vi "pco.camera_Live_ConvertSettings_Example_IMAQ.vi"() -> ()   [LabVIEW 2020]
doc: "A short program to demonstrate the fundamentals of control and image acquision with the pco.camera series. The program records a sequence of images, with \"live\" updating, until the \"StopRecording\" button is pressed. Use ctrl-H for more help on the individual controls and indicators.\n\nCopyright 2004, 2010 The Cooke Corporation."
uses:
  Camera.lvclass
  TimingControl.lvlib
panel:
  in  "settingsChanged":bool
  in  "Trigger":bool
  in  "LUT File":path
  in  "data_format":T1(ring)=enum."RGBA8"
  out "Image":T2(plugin-control)
  in  "Auto Range":bool
  out "rawImage":u16[][](array[numeric])
  in  "iContrast [%]":i32 min=-100 max=99 step=1
  in  "Gamma":dbl=1.0 min=0.01 max=10.0 step=0.01 format="%.2f"
  in  "whiteBalance":bool
  in  "iScale_max":u16=60000 step=1
  in  "iScale_min":u16=200 step=1
  in  "Image Index":u32 max=9
  out "Recorded Images":u32
  in  "TriggerMode":T3(ring)
  in  "Quit":bool
  out "Error":errorcluster {"code" format="%x"}
  in  "Stop Record":bool
  out "Recording On":bool
  in  "roiY1":u64=2 min=1 max=2160 step=1
  in  "roiX1":u64=2 min=1 max=2560 step=1
  in  "roiY0":u64=1 min=1 max=2159 step=1
  in  "roiX0":u64=1 min=1 max=2559 step=1
  out "Image Height":u64
  out "Image Width":u64
  in  "dwImgCount":u32=10 caption="Required Number of Images" max=2397
  in  "Exposure Time [s]":dbl=0.010000000000000002 min=0.0005 max=2.0 step=0.001
  # "This example demonstrates the image acquisition with one camera in ring buffer mode together with a live display of the latest images during record. After record is stopped, the images can be addressed by index.\nAdditionally the image convert settings can be adjusted at any time\nNote that this example will not be fail save, i.e. doesnt react on errors, just handles them forward to the end\n\nUsage:\nSelect your required image count and the camera setup before you start the program.\nOnce started, the camera class will be initialized and images will be recorded and displayed automatically\nYou can stop the images by pressing stop record.\nAfter stopped, the image at the selected index will be read out\nTo finish the program click on quit application, this will force an exit of the camera class\nYou can change your required ROI after and also during the record."
  # "pco.labview"
  # "Camera Setup"
  # "Recording Control"
  # "Parameters for image readout"
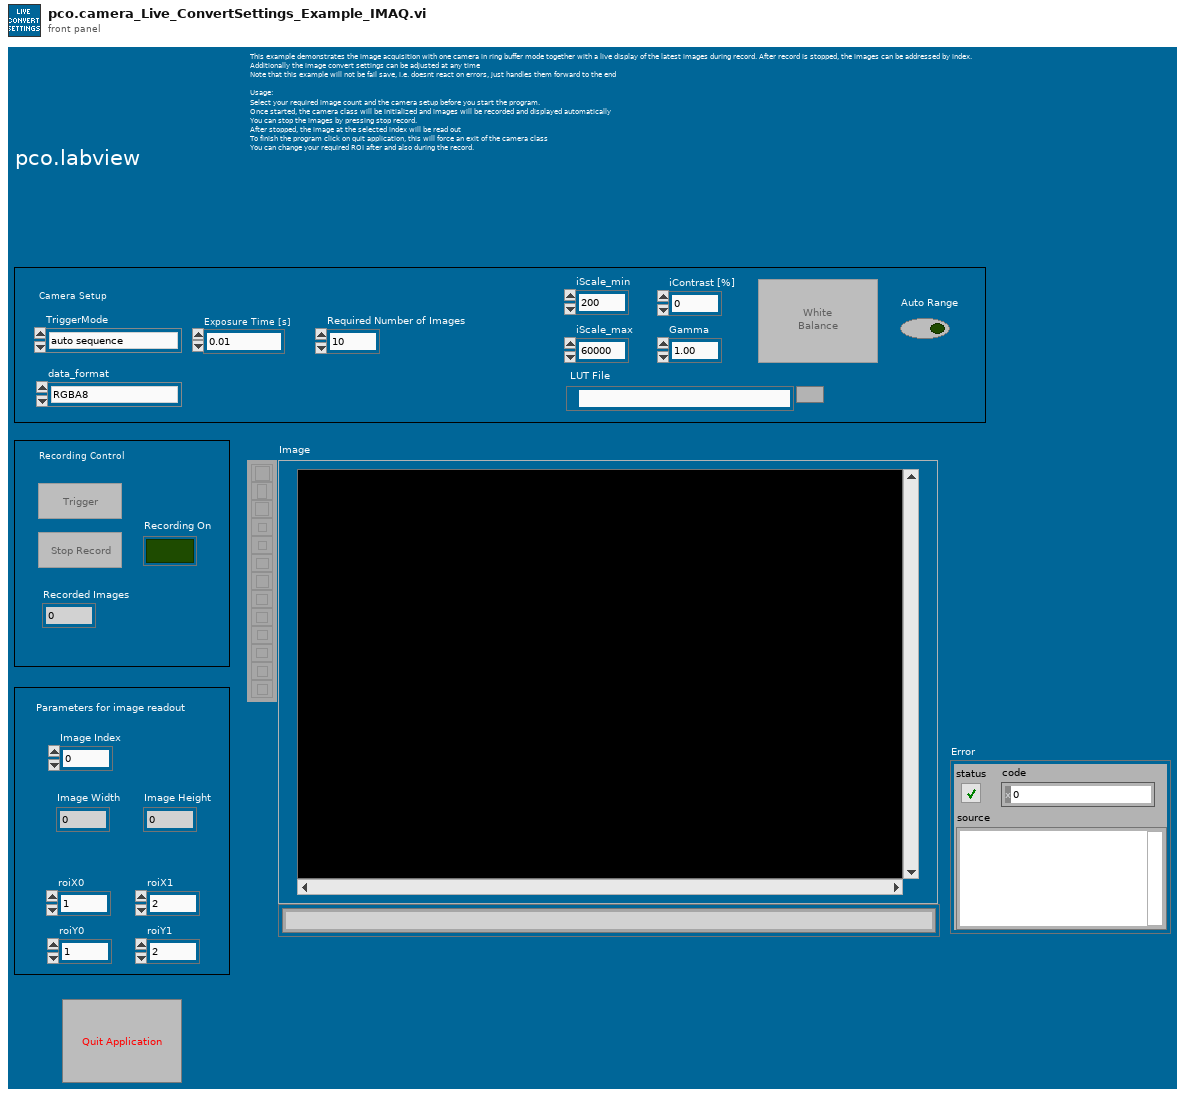
[diagram p1: front panel]
types:
  T1 = enum16{"Undefined", "Mono8", "Mono16", "BGRA8", "RGBA8", "BGRA16", "RGBA16", "CompressedMono8"}
  T2 = typedef "IMAQ Image.ctl" = refnum<image>
  T3 = enum16{"auto sequence", "software trigger", "external exposure start", "external exposure control"}
  T4 = enum16{"sequence", "sequence non blocking", "ring buffer", "fifo", "sequence_dpcore", "sequence_non_blocking_dpcore", "ring_buffer_dpcore", "fifo_dpcore", "tif", "multitif", "pcoraw", "b16", "dicom", "multidicom"}
  T5 = enum8{"Enabled", "Disabled", "Disabled and Grayed Out"}
  T6 = cluster{"serial":u32, "type":u16, "sub_type":u16, "interface_type":u16, "bit_resolution":u16, "min_exposure_time_s":dbl, "max_exposure_time_s":dbl, "min_exposure_step_s":dbl, "min_delay_time_s":dbl, "max_delay_time_s":dbl, "min_delay_step_s":dbl, "min_width":u64, "min_height":u64, "max_width":u64, "max_height":u64, "roi_step_horz":u64, "roi_step_vert":u64, "roi_symmetric_horz":bool, "roi_symmetric_vert":bool, "has_timestamp_mode":bool, "has_timestamp_mode_ascii_only":bool, "pixelrate_vec":u32[], "has_acquire_mode":bool, "has_ext_acquire_mode":bool, "has_metadata_mode":bool, "has_ram":bool, "binning_horz_vec":u16[], "binning_vert_vec":u16[]}
  T7 = typedef "Image Type" = u32
  T8 = typedef "Camera.lvclass/binning.ctl" = cluster{"vert":u16, "horz":u16}
  T9 = cluster{"exposure_time_s":dbl, "delay_time_s":dbl, "roi":cluster{"x0":u64, "y0":u64, "x1":u64, "y1":u64}, "timestamp_mode":u16, "pixelrate":u32, "trigger_mode":u16, "acquire_mode":u16, "metadata_mode":u16, "noisefilter_mode":u16, "binning":T8}
  T10 = cluster{"sharpen":bool, "adaptive_sharpen":bool, "flip_vertical":bool, "auto_minmax":bool, "min_limit":u16, "max_limit":u16, "gamma":dbl, "contrast":i32, "pco_debayer_algorithm":bool, "color_temperature":i32, "color_saturation":i32, "color_vibrance":i32, "color_tint":i32, "lut_file":path}
  T11 = cluster{"Plane 4 (alpha)":u16, "Plane 1 (Red)":u16, "Plane 2 (Green)":u16, "Plane 3 (Blue)":u16}[][]
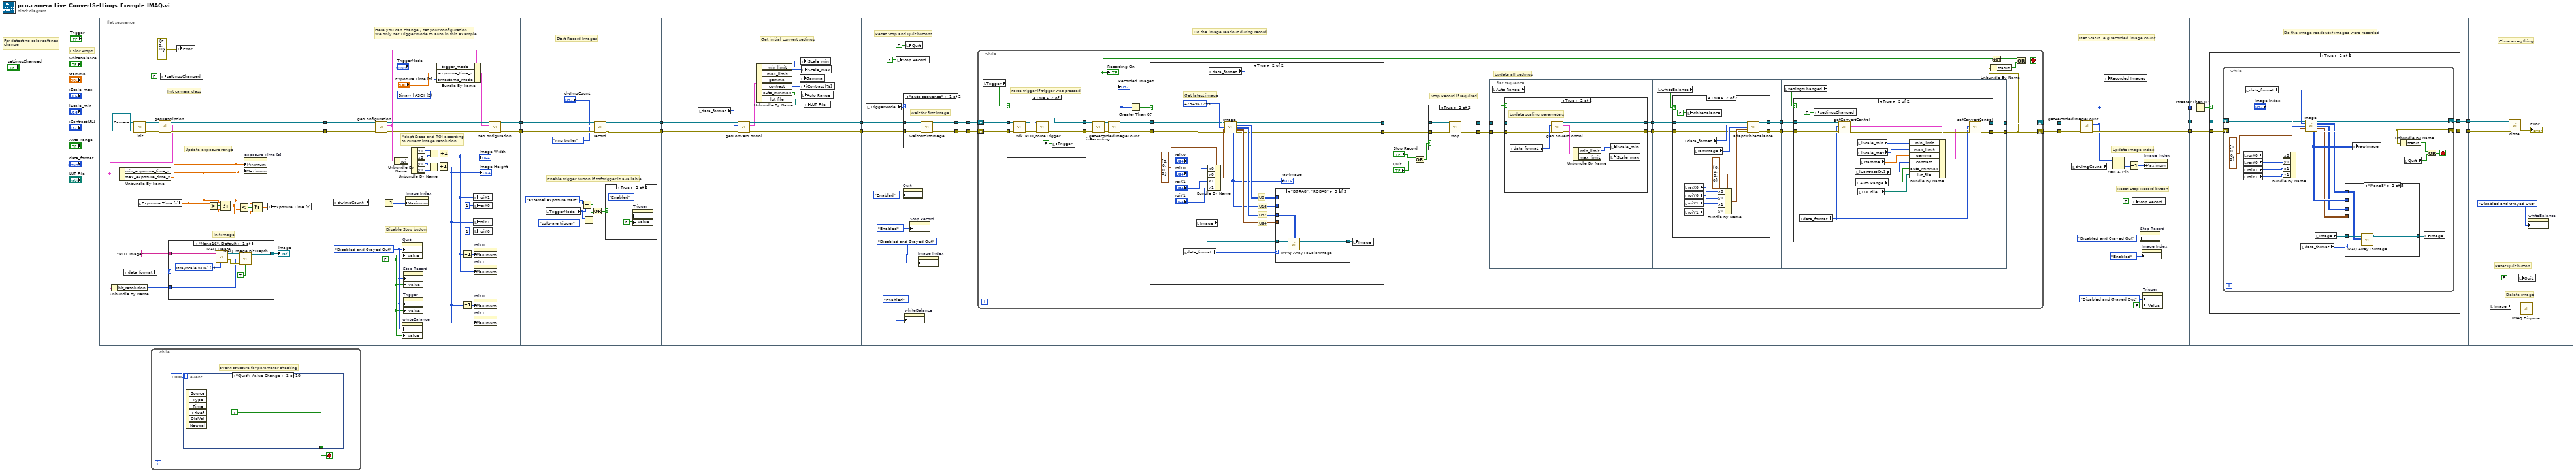
[diagram p0: block diagram]
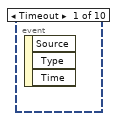
[diagram p2: hidden frame]
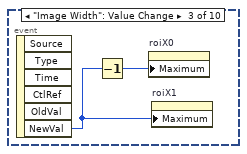
[diagram p3: hidden frame]
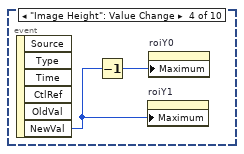
[diagram p4: hidden frame]
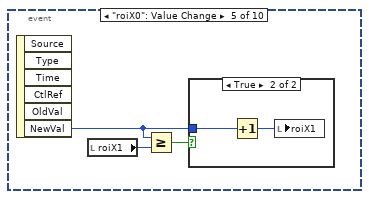
[diagram p5: hidden frame]
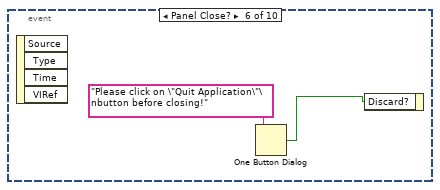
[diagram p7: hidden frame]
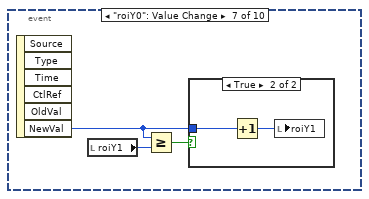
[diagram p8: hidden frame]
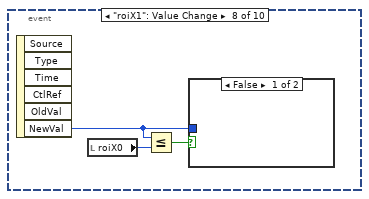
[diagram p10: hidden frame]
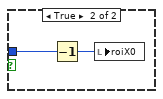
[diagram p11: hidden frame]
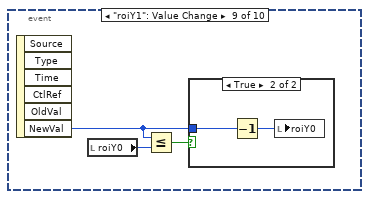
[diagram p12: hidden frame]
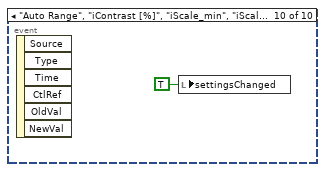
[diagram p14: hidden frame]
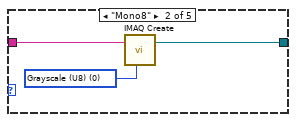
[diagram p15: hidden frame]
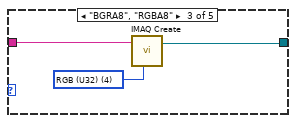
[diagram p16: hidden frame]
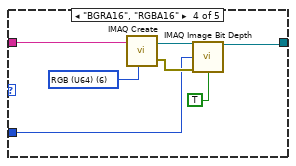
[diagram p17: hidden frame]
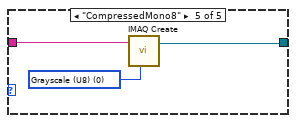
[diagram p18: hidden frame]
diagram:
  # "For detecting color settings\nchange"
  # "Color Props"
  n1 = flat-sequence {
    tunnel: [w25] -> w7
    tunnel: [w24] -> w6
    tunnel: [w64] -> w17
    tunnel: [w68] -> w16
    tunnel: w7 -> [w63]
    tunnel: w6 -> [w62]
    tunnel: w17 -> [w98]
    tunnel: w16 -> [w99]
    tunnel: [w95] -> w11
    tunnel: [w96] -> w8
    tunnel: w11 -> [w112]
    tunnel: [w107] -> w10
    tunnel: [w113] -> w9
    tunnel: w8 -> [w103]
    tunnel: w10 -> [w120]
    tunnel: w9 -> [w121]
    tunnel: [w119] -> w15
    tunnel: [w116] -> w2
    tunnel: w15 -> [w134]
    tunnel: [w133] -> w14
    tunnel: [w132] -> w5
    tunnel: w2 -> [w131]
    tunnel: w14 -> [w281]
    tunnel: [w279] -> w13
    tunnel: w5 -> [w274]
    tunnel: [w273] -> w4
    tunnel: [w272] -> w1
    tunnel: w13 -> [w290]
    tunnel: [w289] -> w12
    tunnel: w4 -> [w288]
    tunnel: [w287] -> w3
    tunnel: w1 -> [w285]
    tunnel: w12 -> [w338]
    tunnel: w3 -> [w335]
    frame #0 {
      # "Init image"
      # "Init camera class"
      # "Update exposure range"
      n2 = local read "data_format"() -> (w21:T1)
      n3 = call-dynamic "init.vi"("Camera in"=refnum<class "Camera.lvclass"> refnum) -> ("Camera out"=w26:refnum<class "Camera.lvclass">, "error out"=w27:errorcluster)  [unwired: 8 in]
      n4 = local read "Exposure Time [s]"() -> (w35:dbl)
      n5 = call-dynamic "getDescription.vi"("error in (no error)"=w27, "Camera in"=w26) -> ("error out"=w24:errorcluster, "description"=w19:T6, "Camera out"=w25:refnum<class "Camera.lvclass">)  [unwired: 7 in]
      n6 = Unbundle By Name(w19) -> ("bit_resolution"=w18:u16)
      n7 = Unbundle By Name(w19) -> ("min_exposure_time_s"=w23:dbl, "max_exposure_time_s"=w22:dbl)
      n8 = local write "settingsChanged"(FALSE ("settingsChanged")) -> ()
      n9 = case shown="\"Mono16\", Default" w21 {
        tunnel: "PCO Image" ("Image Name") -> [w42 w46 w48 w55 w58]
        tunnel: [w38 w44 w47 w51 w57] -> w28
        tunnel: w18 -> [w37 _ _ w50 _]
        frame "Mono16", Default {
          w43 = T7 7 items=["Grayscale (U8)", "Grayscale (I16)", "Grayscale (SGL)", "Complex (CSG)", "RGB (U32)", "HSL (U32)", "RGB (U64)", "Grayscale (U16)"] ("Image Type")
          n10 = call "IMAQ Create"("Image Name"=w42, "Image Type"=w43) -> ("New Image"=w40:T2, "error out"=w39:errorcluster)  [unwired: 3 in]
          n11 = call "IMAQ Image Bit Depth"("Image"=w40, "Bit Depth (0)"=w37, "error in (no error)"=w39, "Get/Set Bit Depth? (Set)"=TRUE) -> ("Image Out"=w38:T2)  [unwired: 9 in, 2 out]
        }
        frame "Mono8" {
          w45 = T7 0 items=["Grayscale (U8)", "Grayscale (I16)", "Grayscale (SGL)", "Complex (CSG)", "RGB (U32)", "HSL (U32)", "RGB (U64)", "Grayscale (U16)"] ("Image Type")
          n12 = call "IMAQ Create"("Image Name"=w46, "Image Type"=w45) -> ("New Image"=w44:T2)  [unwired: 3 in, 1 out]
        }
        frame "BGRA8", "RGBA8" {
          w49 = T7 4 items=["Grayscale (U8)", "Grayscale (I16)", "Grayscale (SGL)", "Complex (CSG)", "RGB (U32)", "HSL (U32)", "RGB (U64)", "Grayscale (U16)"] ("Image Type")
          n13 = call "IMAQ Create"("Image Name"=w48, "Image Type"=w49) -> ("New Image"=w47:T2)  [unwired: 3 in, 1 out]
        }
        frame "BGRA16", "RGBA16" {
          w56 = T7 6 items=["Grayscale (U8)", "Grayscale (I16)", "Grayscale (SGL)", "Complex (CSG)", "RGB (U32)", "HSL (U32)", "RGB (U64)", "Grayscale (U16)"] ("Image Type")
          n14 = call "IMAQ Create"("Image Name"=w55, "Image Type"=w56) -> ("New Image"=w53:T2, "error out"=w52:errorcluster)  [unwired: 3 in]
          n15 = call "IMAQ Image Bit Depth"("Image"=w53, "Bit Depth (0)"=w50, "error in (no error)"=w52, "Get/Set Bit Depth? (Set)"=TRUE) -> ("Image Out"=w51:T2)  [unwired: 9 in, 2 out]
        }
        frame "CompressedMono8" {
          w59 = T7 0 items=["Grayscale (U8)", "Grayscale (I16)", "Grayscale (SGL)", "Complex (CSG)", "RGB (U32)", "HSL (U32)", "RGB (U64)", "Grayscale (U16)"] ("Image Type")
          n16 = call "IMAQ Create"("Image Name"=w58, "Image Type"=w59) -> ("New Image"=w57:T2)  [unwired: 3 in, 1 out]
        }
      }
      "Image" <- w28
      n17 = local write "Error"(errorcluster {"status"=FALSE, "code"=0, "source"=""} ("error IO")) -> ()
      n18 = Greater?(x=w35, y=w22) -> (0:w36:bool)
      n19 = Select(t=w22, s=w36, f=w35) -> (s? t:f=w33:dbl)
      n20 = Less?(x=w33, y=w23) -> (x < y?=w34:bool)
      n21 = property on="Exposure Time [s]" class="DigNum (strict)"("Minimum"=w23, "Maximum"=w22) -> ()  [unwired: 2 in, 2 out]
      n22 = Select(t=w23, s=w34, f=w33) -> (s? t:f=w32:dbl)
      n23 = local write "Exposure Time [s]"(w32) -> ()
    }
    frame #1 {
      w74 = u16 2 items=["OFF", "Binary", "Binary+ASCII", "ASCII"] ("wTimeStampMode")
      w60 = FALSE ("Stop")
      w61 = T5."Disabled and Grayed Out" ("Disabled")
      # "Disable Stop button"
      # "Adapt Sizes and ROI according\nto current image resolution"
      # "Here you can change / set your configuration\nWe only set Trigger mode to auto in this example"
      n24 = local read "dwImgCount"() -> (w75:u32)
      n25 = call-dynamic "getConfiguration.vi"("error in (no error)"=w62, "Camera in"=w63) -> ("error out"=w69:errorcluster, "configuration"=w80:T9, "Camera out"=w71:refnum<class "Camera.lvclass">)  [unwired: 7 in]
      n26 = Decrement(x=w75) -> (x-1=w65:u32)
      n27 = Unbundle By Name(w80) -> ("roi"=w81:cluster{"x0":u64, "y0":u64, "x1":u64, "y1":u64})
      n28 = property on="Quit" class="Bool (strict)"("DisabledEnum"=w61, "Value"=w60) -> ()  [unwired: 2 in, 2 out]
      n29 = property on="whiteBalance" class="Bool (strict)"("DisabledEnum"=w61, "Value"=w60) -> ()  [unwired: 2 in, 2 out]
      n30 = property on="Stop Record" class="Bool (strict)"("DisabledEnum"=w61, "Value"=w60) -> ()  [unwired: 2 in, 2 out]
      n31 = property on="Trigger" class="Bool (strict)"("DisabledEnum"=w61, "Value"=w60) -> ()  [unwired: 2 in, 2 out]
      n32 = property on="Image Index" class="DigNum (strict)"("Maximum"=w65) -> ()  [unwired: 2 in, 2 out]
      n33 = Unbundle By Name(w81) -> ("x1"=w83:u64, "x0"=w82:u64, "y1"=w85:u64, "y0"=w84:u64)
      n34 = Subtract(x=w85, y=w84) -> (x-y=w87:u64)
      n35 = Subtract(x=w83, y=w82) -> (x-y=w86:u64)
      n36 = Bundle By Name(cluster=w80, "trigger_mode"="TriggerMode", "exposure_time_s"="Exposure Time [s]", "timestamp_mode"=w74) -> (w70:T9)
      n37 = Increment(x=w87) -> (x+1=w66:u64)
      "Image Height" <- w66
      n38 = Increment(x=w86) -> (x+1=w67:u64)
      "Image Width" <- w67
      n39 = Decrement(x=w67) -> (x-1=w78:u64)
      n40 = Decrement(x=w66) -> (x-1=w79:u64)
      n41 = local write "roiX1"(w67) -> ()
      n42 = local write "roiX0"(u64 1 ("roiY0")) -> ()
      n43 = local write "roiY1"(w66) -> ()
      n44 = local write "roiY0"(u64 1 ("roiY0")) -> ()
      n45 = property on="roiX0" class="DigNum (strict)"("Maximum"=w78) -> ()  [unwired: 2 in, 2 out]
      n46 = property on="roiX1" class="DigNum (strict)"("Maximum"=w67) -> ()  [unwired: 2 in, 2 out]
      n47 = property on="roiY0" class="DigNum (strict)"("Maximum"=w79) -> ()  [unwired: 2 in, 2 out]
      n48 = property on="roiY1" class="DigNum (strict)"("Maximum"=w66) -> ()  [unwired: 2 in, 2 out]
      n49 = call-dynamic "setConfiguration.vi"("error in (no error)"=w69, "configuration"=w70, "Camera in"=w71) -> ("error out"=w68:errorcluster, "Camera out"=w64:refnum<class "Camera.lvclass">)  [unwired: 7 in]
    }
    frame #2 {
      # "Enable trigger button if softtrigger is available"
      # "Start Record Images"
      n50 = local read "TriggerMode"() -> (w93:T3)
      n51 = Equal?(x=T3."external exposure start" ("TriggerMode"), y=w93) -> (x = y?=w90:bool)
      n52 = Equal?(x=w93, y=T3."software trigger" ("TriggerMode")) -> (x = y?=w89:bool)
      n53 = Or(x=w90, y=w89) -> (x .or. y?=w91:bool)
      n54 = call-dynamic "record.vi"("Camera in"=w98, "num_images"="dwImgCount", "record_mode"=T4."ring buffer", "error in (no error)"=w99) -> ("Camera out"=w96:refnum<class "Camera.lvclass">, "error out"=w95:errorcluster)  [unwired: 10 in]
      n55 = case shown="True" w91 {
        frame False {
        }
        frame True {
          n56 = property on="Trigger" class="Bool (strict)"("DisabledEnum"=T5."Enabled" ("Disabled"), "Value"=FALSE ("Trigger")) -> ()  [unwired: 2 in, 2 out]
        }
      }
    }
    frame #3 {
      # "Get initial convert settings"
      n57 = local read "data_format"() -> (w102:T1)
      n58 = call-dynamic "getConvertControl.vi"("error in (no error)"=w112, "data_format"=w102, "Camera in"=w103) -> ("error out"=w107:errorcluster, "convert_control"=w111:T10, "Camera out"=w113:refnum<class "Camera.lvclass">)  [unwired: 6 in]
      n59 = Unbundle By Name(w111) -> ("min_limit"=w109:u16, "max_limit"=w108:u16, "gamma"=w110:dbl, "contrast"=w106:i32, "auto_minmax"=w105:bool, "lut_file"=w104:path)
      n60 = local write "iContrast [%]"(w106) -> ()
      n61 = local write "Gamma"(w110) -> ()
      n62 = local write "iScale_min"(w109) -> ()
      n63 = local write "iScale_max"(w108) -> ()
      n64 = local write "Auto Range"(w105) -> ()
      n65 = local write "LUT File"(w104) -> ()
    }
    frame #4 {
      # "Reset Stop and Quit buttons"
      n66 = local read "TriggerMode"() -> (w114:T3)
      n67 = local write "Stop Record"(FALSE ("Stop Record")) -> ()
      n68 = case shown="\"auto sequence\"" w114 {
        tunnel: w121 -> [w128 w130]
        tunnel: w120 -> [w127 w129]
        tunnel: [w126 w129] -> w119
        tunnel: [w125 w130] -> w116
        frame "auto sequence" {
          # "Wait for first image"
          n69 = call-dynamic "waitForFirstImage.vi"("error in (no error)"=w127, "Camera in"=w128) -> ("error out"=w126:errorcluster, "Camera out"=w125:refnum<class "Camera.lvclass">)  [unwired: 8 in]
        }
        frame Default {
          # "Don't wait \nif we trigger"
        }
      }
      n70 = property on="Quit" class="Bool (strict)"("DisabledEnum"=T5."Enabled" ("Disabled")) -> ()  [unwired: 2 in, 2 out]
      n71 = property on="whiteBalance" class="Bool (strict)"("DisabledEnum"=T5."Enabled" ("Disabled")) -> ()  [unwired: 2 in, 2 out]
      n72 = local write "Quit"(FALSE ("Stop")) -> ()
      n73 = property on="Stop Record" class="Bool (strict)"("DisabledEnum"=T5."Enabled" ("Disabled")) -> ()  [unwired: 2 in, 2 out]
      n74 = property on="Image Index" class="DigNum (strict)"("DisabledEnum"=T5."Disabled and Grayed Out" ("Disabled")) -> ()  [unwired: 2 in, 2 out]
    }
    frame #5 {
      # "Do the image readout during record"
      n75 = while {
        shift-right: [w144] -> w133
        shift-left: w134 -> [w147]
        shift-right: [w150] -> w132
        shift-left: w131 -> [w148]
        stop <- w162 stop-if-true
        # "Stop Record if required"
        # "Force trigger if trigger was pressed"
        # "Update all settings"
        n76 = local read "Trigger"() -> (w149:bool)
        n77 = case shown="True" w149 {
          tunnel: w148 -> [w206 w211]
          tunnel: w147 -> [w205 w210]
          tunnel: [w206 w209] -> w146
          tunnel: [w205 w208] -> w145
          frame False {
          }
          frame True {
            n78 = call-dynamic "sdk.vi"("Camera in"=w211, "error in (no error)"=w210) -> ("Camera out"=w209:refnum<class "Camera.lvclass">, "sdk"=w212:u64, "error out"=w213:errorcluster)  [unwired: 11 in]
            n79 = call "PCO_ForceTrigger.vi"("error in (no error)"=w213, "ph"=w212) -> ("error out"=w208:errorcluster)  [unwired: 6 in, 3 out]
            n80 = local write "Trigger"(FALSE ("Trigger")) -> ()
          }
        }
        n81 = call-dynamic "isRecording.vi"("Camera in"=w146, "error in (no error)"=w145) -> ("Camera out"=w158:refnum<class "Camera.lvclass">, "recording"=w160:bool, "error out"=w157:errorcluster)  [unwired: 11 in]
        "Recording On" <- w160
        n82 = call-dynamic "getRecordedImageCount.vi"("Camera in"=w158, "error in (no error)"=w157) -> ("Camera out"=w155:refnum<class "Camera.lvclass">, "recorded_image_count"=w143:u32, "error out"=w156:errorcluster)  [unwired: 11 in]
        "Recorded Images" <- w143
        n83 = Greater Than 0?(x=w143) -> (x > 0?=w142:bool)
        n84 = case shown="True" w142 {
          tunnel: w156 -> [w169 w182]
          tunnel: w155 -> [w170 w173]
          tunnel: [w169 w171] -> w138
          tunnel: [w170 w172] -> w137
          frame False {
          }
          frame True {
            # "U64"
            # "U32"
            # "U8"
            # "U16"
            # "Get latest image"
            n85 = local read "data_format"() -> (w174:T1)
            n86 = local read "Image"() -> (w179:T2)
            n87 = Bundle By Name(cluster=cluster{"x0":u64, "y0":u64, "x1":u64, "y1":u64} {"x0"=0, "y0"=0, "x1"=0, "y1"=0} ("roi"), "x0"="roiX0", "y0"="roiY0", "x1"="roiX1", "y1"="roiY1") -> (w185:cluster{"x0":u64, "y0":u64, "x1":u64, "y1":u64})
            n88 = local read "data_format"() -> (w181:T1)
            n89 = call-dynamic "image.vi"("Camera in"=w173, "data_format"=w181, "image_index"=u32 4294967295 ("dwImgIdx"), "roi"=w185, "error in (no error)"=w182) -> ("Camera out"=w172:refnum<class "Camera.lvclass">, "image (U8)"=w176:u8[][], "image (U32)"=w177:u32[][], "image (U64)"=w178:T11, "raw_image (U16)"=w175:u16[][], "error out"=w171:errorcluster)  [unwired: 3 in, 2 out]
            "rawImage" <- w175
            n90 = case shown="\"BGRA8\", \"RGBA8\"" w174 {
              tunnel: w179 -> [w192 w195 w198 w201 w204]
              tunnel: [w190 w193 w197 w199 w203] -> w180
              tunnel: w178 -> [_ _ _ w200 _]
              tunnel: w177 -> [_ _ w196 _ _]
              tunnel: w176 -> [_ w194 _ _ w202]
              tunnel: w175 -> [w191 _ _ _ _]
              frame "Mono16", Default {
                n91 = call "IMAQ ArrayToImage"("Image Pixels (U16)"=w191, "Image"=w192) -> ("Image Out"=w190:T2)  [unwired: 8 in, 1 out]
              }
              frame "Mono8" {
                n92 = call "IMAQ ArrayToImage"("Image Pixels (U8)"=w194, "Image"=w195) -> ("Image Out"=w193:T2)  [unwired: 8 in, 1 out]
              }
              frame "BGRA8", "RGBA8" {
                n93 = call "IMAQ ArrayToColorImage"("Image Pixels (U32)"=w196, "Image"=w198) -> ("Image Out"=w197:T2)  [unwired: 3 in, 1 out]
              }
              frame "BGRA16", "RGBA16" {
                n94 = call "IMAQ ArrayToColorImage"("Image"=w201, "Image Pixels (U64)"=w200) -> ("Image Out"=w199:T2)  [unwired: 3 in, 1 out]
              }
              frame "CompressedMono8" {
                n95 = call "IMAQ ArrayToImage"("Image Pixels (U8)"=w202, "Image"=w204) -> ("Image Out"=w203:T2)  [unwired: 8 in, 1 out]
              }
            }
            n96 = local write "Image"(w180) -> ()
          }
        }
        n97 = Or(x="Stop Record", y="Quit") -> (x .or. y?=w141:bool)
        n98 = case shown="True" w141 {
          tunnel: w138 -> [w164 w165]
          tunnel: [w163 w167] -> w136
          tunnel: [w164 w168] -> w135
          tunnel: w137 -> [w163 w166]
          frame False {
          }
          frame True {
            n99 = call-dynamic "stop.vi"("error in (no error)"=w165, "Camera in"=w166) -> ("error out"=w168:errorcluster, "Camera out"=w167:refnum<class "Camera.lvclass">)  [unwired: 8 in]
          }
        }
        n100 = flat-sequence {
          tunnel: w135 -> [w216]
          tunnel: w136 -> [w217]
          tunnel: [w215] -> w154
          tunnel: [w214] -> w153
          tunnel: w154 -> [w232]
          tunnel: w153 -> [w231]
          tunnel: [w230] -> w152
          tunnel: [w229] -> w151
          tunnel: w152 -> [w251]
          tunnel: w151 -> [w252]
          tunnel: [w250] -> w144
          tunnel: [w249] -> w150
          frame #0 {
            n101 = local read "Auto Range"() -> (w218:bool)
            n102 = case shown="True" w218 {
              tunnel: w217 -> [w220 w224]
              tunnel: w216 -> [w219 w223]
              tunnel: [w219 w222] -> w215
              tunnel: [w220 w221] -> w214
              frame False {
              }
              frame True {
                # "Update scaling parameters"
                n103 = local read "data_format"() -> (w228:T1)
                n104 = call-dynamic "getConvertControl.vi"("error in (no error)"=w223, "data_format"=w228, "Camera in"=w224) -> ("error out"=w222:errorcluster, "convert_control"=w225:T10, "Camera out"=w221:refnum<class "Camera.lvclass">)  [unwired: 6 in]
                n105 = Unbundle By Name(w225) -> ("min_limit"=w226:u16, "max_limit"=w227:u16)
                n106 = local write "iScale_max"(w227) -> ()
                n107 = local write "iScale_min"(w226) -> ()
              }
            }
          }
          frame #1 {
            n108 = local read "whiteBalance"() -> (w233:bool)
            n109 = case shown="True" w233 {
              tunnel: w232 -> [w234 w240]
              tunnel: w231 -> [w235 w239]
              tunnel: [w234 w238] -> w230
              tunnel: [w235 w237] -> w229
              frame False {
              }
              frame True {
                n110 = local read "data_format"() -> (w247:T1)
                n111 = local read "roiX0"() -> (w245:u64)
                n112 = local read "roiY0"() -> (w244:u64)
                n113 = local read "roiX1"() -> (w243:u64)
                n114 = local read "roiY1"() -> (w236:u64)
                n115 = local write "whiteBalance"(FALSE ("whiteBalance")) -> ()
                n116 = local read "rawImage"() -> (w246:u16[][])
                n117 = Bundle By Name(cluster=cluster{"x0":u64, "y0":u64, "x1":u64, "y1":u64} {"x0"=0, "y0"=0, "x1"=0, "y1"=0} ("roi"), "x0"=w245, "y0"=w244, "x1"=w243, "y1"=w236) -> (w242:cluster{"x0":u64, "y0":u64, "x1":u64, "y1":u64})
                n118 = call-dynamic "adaptWhiteBalance.vi"("Camera in"=w239, "data_format"=w247, "raw_image (U16)"=w246, "roi"=w242, "error in (no error)"=w240) -> ("Camera out"=w237:refnum<class "Camera.lvclass">, "error out"=w238:errorcluster)  [unwired: 9 in]
              }
            }
          }
          frame #2 {
            n119 = local read "settingsChanged"() -> (w253:bool)
            n120 = case shown="True" w253 {
              tunnel: w252 -> [w255 w261]
              tunnel: w251 -> [w254 w260]
              tunnel: [w254 w257] -> w250
              tunnel: [w255 w256] -> w249
              frame False {
              }
              frame True {
                n121 = local read "data_format"() -> (w259:T1)
                n122 = local write "settingsChanged"(FALSE ("whiteBalance")) -> ()
                n123 = call-dynamic "getConvertControl.vi"("error in (no error)"=w260, "data_format"=w259, "Camera in"=w261) -> ("error out"=w263:errorcluster, "convert_control"=w270:T10, "Camera out"=w264:refnum<class "Camera.lvclass">)  [unwired: 6 in]
                n124 = local read "iContrast [%]"() -> (w266:i32)
                n125 = local read "Auto Range"() -> (w265:bool)
                n126 = local read "iScale_min"() -> (w269:u16)
                n127 = local read "iScale_max"() -> (w268:u16)
                n128 = local read "LUT File"() -> (w258:path)
                n129 = local read "Gamma"() -> (w267:dbl)
                n130 = Bundle By Name(cluster=w270, "min_limit"=w269, "max_limit"=w268, "gamma"=w267, "contrast"=w266, "auto_minmax"=w265, "lut_file"=w258) -> (w262:T10)
                n131 = call-dynamic "setConvertControl.vi"("error in (no error)"=w263, "convert_control"=w262, "data_format"=w259, "Camera in"=w264) -> ("error out"=w257:errorcluster, "Camera out"=w256:refnum<class "Camera.lvclass">)  [unwired: 6 in]
              }
            }
          }
        }
        n132 = Unbundle By Name(w144) -> ("status"=w161:bool)
        n133 = Not(x=w160) -> (.not. x?=w159:bool)
        n134 = Or(x=w159, y=w161) -> (x .or. y?=w162:bool)
      }
    }
    frame #6 {
      # "Update image index"
      # "Reset Stop Record button"
      # "Get Status, e.g recorded image count"
      n135 = local read "dwImgCount"() -> (w280:u32)
      n136 = call-dynamic "getRecordedImageCount.vi"("Camera in"=w274, "error in (no error)"=w281) -> ("Camera out"=w273:refnum<class "Camera.lvclass">, "recorded_image_count"=w272:u32, "error out"=w279:errorcluster)  [unwired: 11 in]
      n137 = local write "Recorded Images"(w272) -> ()
      n138 = Max & Min(x=w272, y=w280) -> (min(x,y)=w282:u32)  [unwired: 1 out]
      n139 = Decrement(x=w282) -> (x-1=w277:u32)
      n140 = local write "Stop Record"(FALSE ("Stop Record")) -> ()
      n141 = property on="Stop Record" class="Bool (strict)"("DisabledEnum"=T5."Disabled and Grayed Out" ("Disabled")) -> ()  [unwired: 2 in, 2 out]
      n142 = property on="Image Index" class="DigNum (strict)"("DisabledEnum"=T5."Enabled" ("Disabled")) -> ()  [unwired: 2 in, 2 out]
      n143 = property on="Trigger" class="Bool (strict)"("DisabledEnum"=T5."Disabled and Grayed Out" ("Disabled"), "Value"=FALSE ("Trigger")) -> ()  [unwired: 2 in, 2 out]
      n144 = property on="Image Index" class="DigNum (strict)"("Maximum"=w277) -> ()  [unwired: 2 in, 2 out]
    }
    frame #7 {
      # "Do the image readout if images were recorded"
      n145 = Greater Than 0?(x=w285) -> (x > 0?=w286:bool)
      n146 = case shown="True" w286 {
        tunnel: w290 -> [w291 w296]
        tunnel: [w291 w295] -> w289
        tunnel: w288 -> [w292 w294]
        tunnel: [w292 w293] -> w287
        frame False {
        }
        frame True {
          n147 = while {
            shift-right: [w310] -> w295
            shift-left: w296 -> [w318]
            shift-right: [w297] -> w293
            shift-left: w294 -> [w298]
            stop <- w312 stop-if-true
            n148 = local read "roiX0"() -> (w308:u64)
            n149 = local read "roiY0"() -> (w309:u64)
            n150 = local read "roiX1"() -> (w316:u64)
            n151 = local read "roiY1"() -> (w315:u64)
            n152 = local read "data_format"() -> (w306:T1)
            n153 = Bundle By Name(cluster=cluster{"x0":u64, "y0":u64, "x1":u64, "y1":u64} {"x0"=0, "y0"=0, "x1"=0, "y1"=0} ("roi"), "x0"=w308, "y0"=w309, "x1"=w316, "y1"=w315) -> (w317:cluster{"x0":u64, "y0":u64, "x1":u64, "y1":u64})
            n154 = local read "data_format"() -> (w299:T1)
            n155 = call-dynamic "image.vi"("Camera in"=w298, "data_format"=w306, "image_index"="Image Index", "roi"=w317, "error in (no error)"=w318) -> ("Camera out"=w297:refnum<class "Camera.lvclass">, "image (U8)"=w302:u8[][], "image (U32)"=w301:u32[][], "image (U64)"=w300:T11, "raw_image (U16)"=w303:u16[][], "error out"=w310:errorcluster)  [unwired: 3 in, 2 out]
            n156 = local read "Image"() -> (w304:T2)
            n157 = case shown="\"Mono8\"" w299 {
              tunnel: w304 -> [w321 w324 w327 w330 w333]
              tunnel: [w319 w322 w326 w328 w332] -> w305
              tunnel: w300 -> [_ _ _ w329 _]
              tunnel: w301 -> [_ _ w325 _ _]
              tunnel: w302 -> [_ w323 _ _ w331]
              tunnel: w303 -> [w320 _ _ _ _]
              frame "Mono16", Default {
                n158 = call "IMAQ ArrayToImage"("Image Pixels (U16)"=w320, "Image"=w321) -> ("Image Out"=w319:T2)  [unwired: 8 in, 1 out]
              }
              frame "Mono8" {
                n159 = call "IMAQ ArrayToImage"("Image Pixels (U8)"=w323, "Image"=w324) -> ("Image Out"=w322:T2)  [unwired: 8 in, 1 out]
              }
              frame "BGRA8", "RGBA8" {
                n160 = call "IMAQ ArrayToColorImage"("Image Pixels (U32)"=w325, "Image"=w327) -> ("Image Out"=w326:T2)  [unwired: 3 in, 1 out]
              }
              frame "BGRA16", "RGBA16" {
                n161 = call "IMAQ ArrayToColorImage"("Image"=w330, "Image Pixels (U64)"=w329) -> ("Image Out"=w328:T2)  [unwired: 3 in, 1 out]
              }
              frame "CompressedMono8" {
                n162 = call "IMAQ ArrayToImage"("Image Pixels (U8)"=w331, "Image"=w333) -> ("Image Out"=w332:T2)  [unwired: 8 in, 1 out]
              }
            }
            n163 = local write "rawImage"(w303) -> ()
            n164 = Unbundle By Name(w310) -> ("status"=w313:bool)
            n165 = local read "Quit"() -> (w314:bool)
            n166 = local write "Image"(w305) -> ()
            n167 = Or(x=w313, y=w314) -> (x .or. y?=w312:bool)
          }
        }
      }
    }
    frame #8 {
      # "Delete image"
      # "Close everything"
      # "Reset Quit button"
      n168 = local read "Image"() -> (w334:T2)
      n169 = call-dynamic "close.vi"("error in (no error)"=w338, "Camera in"=w335) -> ("error out"=→"Error":errorcluster)  [unwired: 9 in]
      n170 = local write "Quit"(FALSE ("Stop Record")) -> ()
      n171 = call "IMAQ Dispose"("Image"=w334) -> ()  [unwired: 5 in, 1 out]
      n172 = property on="whiteBalance" class="Bool (strict)"("DisabledEnum"=T5."Disabled and Grayed Out" ("Disabled")) -> ()  [unwired: 2 in, 2 out]
    }
  }
  n173 = while {
    stop <- w340 stop-if-true
    # "Event structure for parameter checking"
    n174 = event shown="[1] \"Quit\": Value Change" {
      selector: _ -> [_ _ _ _ _ _ _ _ _ _]
      dyn-events: _ -> [_ _ _ _ _ _ _ _ _ _]
      timeout: 1000 -> [_ _ _ _ _ _ _ _ _ _]
      tunnel: [_ TRUE _ _ _ _ _ _ _ _] -> w340
      event Timeout {
        n175 = event-data() -> ()  [unwired: 1 in, 3 out]
      }
      event "Quit": Value Change {
        n176 = event-data() -> ()  [unwired: 1 in, 6 out]
      }
      event "Image Width": Value Change {
        n177 = event-data() -> ("NewVal"=w343:u64)  [unwired: 1 in, 5 out]
        n178 = Decrement(x=w343) -> (x-1=w344:u64)
        n179 = property on="roiX0" class="DigNum (strict)"("Maximum"=w344) -> ()  [unwired: 2 in, 2 out]
        n180 = property on="roiX1" class="DigNum (strict)"("Maximum"=w343) -> ()  [unwired: 2 in, 2 out]
      }
      event "Image Height": Value Change {
        n181 = event-data() -> ("NewVal"=w345:u64)  [unwired: 1 in, 5 out]
        n182 = Decrement(x=w345) -> (x-1=w346:u64)
        n183 = property on="roiY1" class="DigNum (strict)"("Maximum"=w345) -> ()  [unwired: 2 in, 2 out]
        n184 = property on="roiY0" class="DigNum (strict)"("Maximum"=w346) -> ()  [unwired: 2 in, 2 out]
      }
      event "roiX0": Value Change {
        n185 = event-data() -> ("NewVal"=w347:u64)  [unwired: 1 in, 5 out]
        n186 = local read "roiX1"() -> (w349:u64)
        n187 = Greater Or Equal?(x=w347, y=w349) -> (x >= y?=w348:bool)
        n188 = case shown="True" w348 {
          tunnel: w347 -> [_ w351]
          frame False {
          }
          frame True {
            n189 = Increment(x=w351) -> (x+1=w350:u64)
            n190 = local write "roiX1"(w350) -> ()
          }
        }
      }
      event Panel Close? {
        n191 = event-data() -> ()  [unwired: 1 in, 4 out]
        n192 = One Button Dialog(message="Please click on \"Quit Application\"\nbutton before closing!") -> (true=w352:bool)  [unwired: 1 in]
        n193 = event-data("Discard?"=w352) -> ()  [unwired: 1 in, 1 out]
      }
      event "roiY0": Value Change {
        n194 = event-data() -> ("NewVal"=w354:u64)  [unwired: 1 in, 5 out]
        n195 = local read "roiY1"() -> (w356:u64)
        n196 = Greater Or Equal?(x=w354, y=w356) -> (x >= y?=w355:bool)
        n197 = case shown="True" w355 {
          tunnel: w354 -> [_ w358]
          frame False {
          }
          frame True {
            n198 = Increment(x=w358) -> (x+1=w357:u64)
            n199 = local write "roiY1"(w357) -> ()
          }
        }
      }
      event "roiX1": Value Change {
        n200 = event-data() -> ("NewVal"=w359:u64)  [unwired: 1 in, 5 out]
        n201 = local read "roiX0"() -> (w361:u64)
        n202 = Less Or Equal?(x=w359, y=w361) -> (x <= y?=w360:bool)
        n203 = case shown="False" w360 {
          tunnel: w359 -> [_ w363]
          frame False {
          }
          frame True {
            n204 = Decrement(x=w363) -> (x-1=w362:u64)
            n205 = local write "roiX0"(w362) -> ()
          }
        }
      }
      event "roiY1": Value Change {
        n206 = event-data() -> ("NewVal"=w364:u64)  [unwired: 1 in, 5 out]
        n207 = local read "roiY0"() -> (w366:u64)
        n208 = Less Or Equal?(x=w364, y=w366) -> (x <= y?=w365:bool)
        n209 = case shown="True" w365 {
          tunnel: w364 -> [_ w368]
          frame False {
          }
          frame True {
            n210 = Decrement(x=w368) -> (x-1=w367:u64)
            n211 = local write "roiY0"(w367) -> ()
          }
        }
      }
      event "Auto Range", "iContrast [%]", "iScale_min", "iScale_max", "Gamma", "LUT File": Value Change {
        n212 = event-data() -> ()  [unwired: 1 in, 6 out]
        n213 = local write "settingsChanged"(TRUE ("settingsChanged")) -> ()
      }
    }
  }
